vi "Get References and Set TEMP FP Labels.vi"(8 "error in":errorcluster, 11 "owner VI":refnum<vi>) -> (0 "error out":errorcluster, 1 "controls found":i32, 3 "owner VI out":refnum<vi>)   [LabVIEW 2024]
doc: "Create a bunch of front panel free labels that will describe the UI Theme Level and Boolean Type for all FP controls->the labels will co-locate with the control so that they can be easily found.\n\n<b>Code Developed By:</b>\nTechnology Service Corporation\n1983 S Liberty Drive\nBloomington, IN 47403\nPhone: 812 558-7100\nwww.tsc.com/atcs"
uses:
  <vilib>/Utility/traverseref.llb/TRef TravTarget.ctl
  <vilib>/Utility/traverseref.llb/VI Scripting - Traverse.lvlib
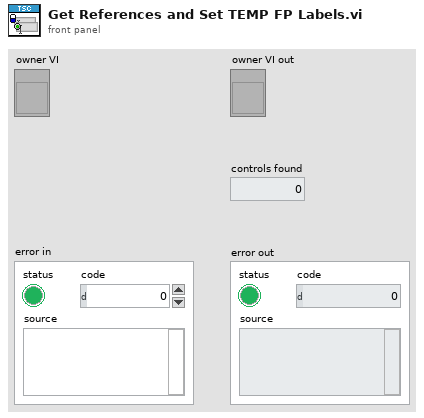
[diagram p1: front panel]
types:
  T1 = typedef "TRef TravTarget.ctl" = enum16{"FP", "BD", "Other"}
  T2 = typedef "LVPositionTypeDef.ctl" = cluster{"Left":i32, "Top":i32}
  T3 = typedef "LVBoundsTypeDef.ctl" = cluster{"Width":u32, "Height":u32}
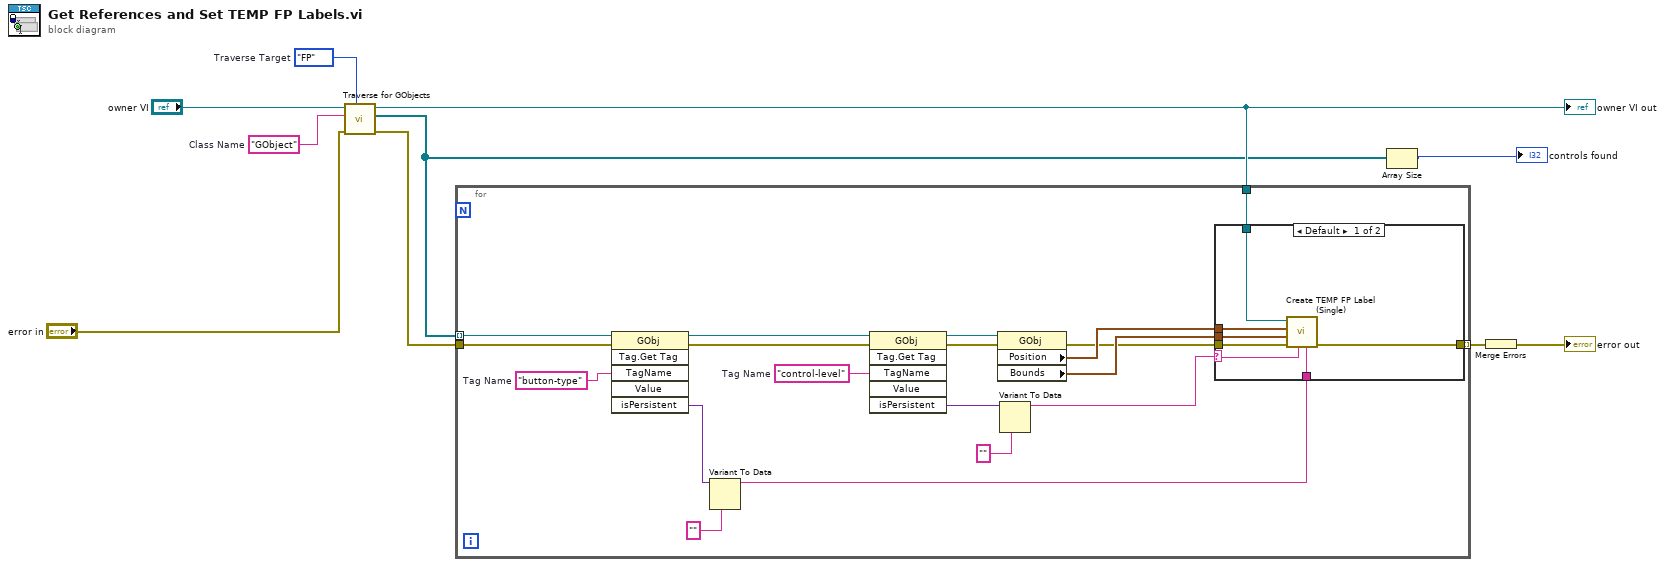
[diagram p0: block diagram]
diagram:
  w9 = TRef_TravTarget."FP"  # Traverse Target
  w10 = "GObject"  # Class Name
  n1 = call <vilib>:"Traverse for GObjects.vi"("Traverse Target"=w9, "error in (no error)"="error in", "Class Name"=w10, "VI Refnum"="owner VI") -> ("error out"=w8:errorcluster, "References"=w2:refnum<vi>[], "dup VI Refnum"=w3:refnum<vi>)  [unwired: 4 in, 1 out]
  "owner VI out" <- w3
  n2 = for {
    tunnel: w2 -> [w28] mode=indexing
    tunnel: w8 -> [w25]
    tunnel: w3 -> [w22]
    tunnel: [w19] -> w7 mode=indexing
    w12 = "control-level"  # Tag Name
    w29 = "button-type"  # Tag Name
    n3 = invoke class="GObj" method="Tag.Get Tag"(reference=w28, error in=w25, "TagName"=w29) -> (reference out=w17:refnum<vi>, error out=w24:errorcluster, "isPersistent"=w27:variant)  [unwired: 3 in, 3 out]
    n4 = Variant To Data(type="", Variant=w27) -> (data=w11:string)  [unwired: 1 in, 1 out]
    n5 = invoke class="GObj" method="Tag.Get Tag"(reference=w17, error in=w24, "TagName"=w12) -> (reference out=w16:refnum<vi>, error out=w18:errorcluster, "isPersistent"=w14:variant)  [unwired: 3 in, 3 out]
    n6 = property class="GObj"(reference=w16, error in=w18) -> (error out=w20:errorcluster, "Position"=w23:T2, "Bounds"=w21:T3)  [unwired: 1 out]
    n7 = Variant To Data(type="", Variant=w14) -> (data=w13:string)  [unwired: 1 in, 1 out]
    n8 = case shown="Default" w13 {
      selector: w13 -> [w31 _]
      tunnel: w23 -> [w36 _]
      tunnel: w22 -> [w35 _]
      tunnel: w21 -> [w34 _]
      tunnel: w20 -> [w33 _]
      tunnel: [w32 _] -> w19
      tunnel: w11 -> [w30 _]
      frame Default {
        n9 = call "Create TEMP FP Label (Single).vi"("button type"=w30, "UI theme level"=w31, "error in (no error)"=w33, "Bounds"=w34, "Position"=w36, "owner VI"=w35) -> ("error out"=w32:errorcluster)  [unwired: 5 in]
      }
      frame "" {
      }
    }
  }
  n10 = Array Size(array=w2) -> (size(s)=→"controls found":i32)
  n11 = Merge Errors(w7) -> (→"error out":errorcluster)
